vi "aToAchar.vi"(1 "old char":dbl) -> (0 "new char":dbl)   [LabVIEW 2011]
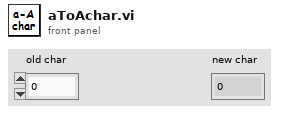
[diagram p1: front panel]
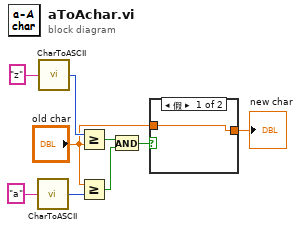
[diagram p0: block diagram]
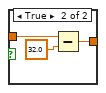
[diagram p2: hidden frame]
diagram:
  n1 = call "CharToASCII.vi"("Character"="a") -> ("ASCII Code"=w8:u8)
  n2 = call "CharToASCII.vi"("Character"="z") -> ("ASCII Code"=w6:u8)
  n3 = Greater Or Equal?(x=w6, y="old char") -> (x >= y?=w5:bool)
  n4 = Greater Or Equal?(x="old char", y=w8) -> (x >= y?=w4:bool)
  n5 = And(x=w5, y=w4) -> (x .and. y?=w3:bool)
  n6 = case shown="假" w3 {
    tunnel: "old char" -> [w10 w13]
    tunnel: [w10 w11] -> w1
    frame False {
    }
    frame True {
      n7 = Subtract(x=w13, y=32.0) -> (x-y=w11:dbl)
    }
  }
  "new char" <- w1
